vi "Serial Number Generator.vi"() -> (3 "UUT Serial #":string)   [LabVIEW 2018]
doc: "Generate a random serial number."
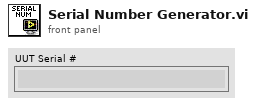
[diagram p1: front panel]
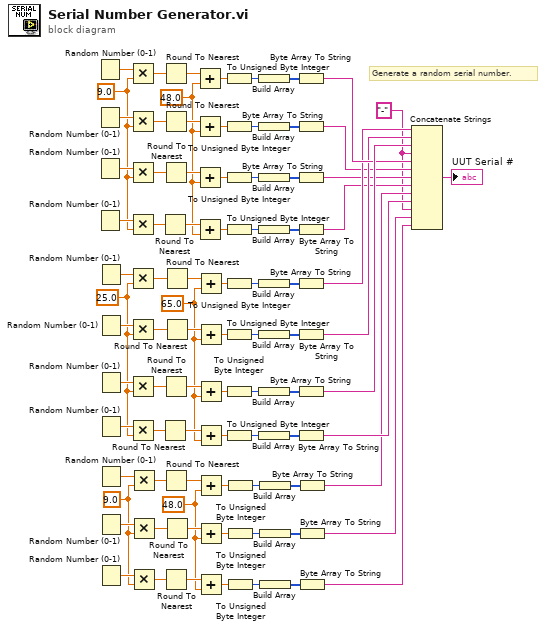
[diagram p0: block diagram]
diagram:
  w1 = 48.0
  w2 = 65.0
  w3 = 48.0
  w6 = 9.0
  w7 = 25.0
  w8 = 9.0
  w4 = "-" ("Substring")
  # "Generate a random serial number."
  n1 = Random Number (0-1)() -> (number: 0 to 1=w9:dbl)
  n2 = Random Number (0-1)() -> (number: 0 to 1=w54:dbl)
  n3 = Random Number (0-1)() -> (number: 0 to 1=w48:dbl)
  n4 = Random Number (0-1)() -> (number: 0 to 1=w42:dbl)
  n5 = Random Number (0-1)() -> (number: 0 to 1=w81:dbl)
  n6 = Random Number (0-1)() -> (number: 0 to 1=w68:dbl)
  n7 = Random Number (0-1)() -> (number: 0 to 1=w67:dbl)
  n8 = Random Number (0-1)() -> (number: 0 to 1=w57:dbl)
  n9 = Random Number (0-1)() -> (number: 0 to 1=w25:dbl)
  n10 = Random Number (0-1)() -> (number: 0 to 1=w30:dbl)
  n11 = Random Number (0-1)() -> (number: 0 to 1=w36:dbl)
  n12 = Multiply(x=w9, y=w8) -> (x*y=w80:dbl)
  n13 = Multiply(x=w54, y=w8) -> (x*y=w55:dbl)
  n14 = Multiply(x=w48, y=w8) -> (x*y=w49:dbl)
  n15 = Multiply(x=w42, y=w8) -> (x*y=w41:dbl)
  n16 = Multiply(x=w81, y=w7) -> (x*y=w79:dbl)
  n17 = Multiply(x=w68, y=w7) -> (x*y=w69:dbl)
  n18 = Multiply(x=w67, y=w7) -> (x*y=w66:dbl)
  n19 = Multiply(x=w57, y=w7) -> (x*y=w58:dbl)
  n20 = Multiply(x=w25, y=w6) -> (x*y=w26:dbl)
  n21 = Multiply(x=w30, y=w6) -> (x*y=w29:dbl)
  n22 = Multiply(x=w36, y=w6) -> (x*y=w35:dbl)
  n23 = Round To Nearest(number=w41) -> (nearest integer value=w17:dbl)
  n24 = Round To Nearest(number=w58) -> (nearest integer value=w13:dbl)
  n25 = Round To Nearest(number=w80) -> (nearest integer value=w20:dbl)
  n26 = Round To Nearest(number=w55) -> (nearest integer value=w19:dbl)
  n27 = Round To Nearest(number=w49) -> (nearest integer value=w18:dbl)
  n28 = Round To Nearest(number=w66) -> (nearest integer value=w14:dbl)
  n29 = Round To Nearest(number=w26) -> (nearest integer value=w12:dbl)
  n30 = Round To Nearest(number=w35) -> (nearest integer value=w10:dbl)
  n31 = Round To Nearest(number=w79) -> (nearest integer value=w16:dbl)
  n32 = Round To Nearest(number=w69) -> (nearest integer value=w15:dbl)
  n33 = Round To Nearest(number=w29) -> (nearest integer value=w11:dbl)
  n34 = Add(x=w20, y=w3) -> (x+y=w78:dbl)
  n35 = Add(x=w19, y=w3) -> (x+y=w56:dbl)
  n36 = Add(x=w18, y=w3) -> (x+y=w50:dbl)
  n37 = Add(x=w17, y=w3) -> (x+y=w40:dbl)
  n38 = Add(x=w16, y=w2) -> (x+y=w74:dbl)
  n39 = Add(x=w15, y=w2) -> (x+y=w73:dbl)
  n40 = Add(x=w14, y=w2) -> (x+y=w63:dbl)
  n41 = Add(x=w13, y=w2) -> (x+y=w62:dbl)
  n42 = Add(x=w12, y=w1) -> (x+y=w27:dbl)
  n43 = Add(x=w11, y=w1) -> (x+y=w28:dbl)
  n44 = Add(x=w10, y=w1) -> (x+y=w34:dbl)
  n45 = To Unsigned Byte Integer(number=w78) -> (unsigned 8bit integer=w83:u8)
  n46 = To Unsigned Byte Integer(number=w56) -> (unsigned 8bit integer=w52:u8)
  n47 = To Unsigned Byte Integer(number=w50) -> (unsigned 8bit integer=w46:u8)
  n48 = To Unsigned Byte Integer(number=w40) -> (unsigned 8bit integer=w43:u8)
  n49 = To Unsigned Byte Integer(number=w74) -> (unsigned 8bit integer=w76:u8)
  n50 = To Unsigned Byte Integer(number=w73) -> (unsigned 8bit integer=w71:u8)
  n51 = To Unsigned Byte Integer(number=w63) -> (unsigned 8bit integer=w65:u8)
  n52 = To Unsigned Byte Integer(number=w62) -> (unsigned 8bit integer=w60:u8)
  n53 = To Unsigned Byte Integer(number=w27) -> (unsigned 8bit integer=w23:u8)
  n54 = To Unsigned Byte Integer(number=w28) -> (unsigned 8bit integer=w32:u8)
  n55 = To Unsigned Byte Integer(number=w34) -> (unsigned 8bit integer=w38:u8)
  n56 = Build Array(w83) -> (w84:u8[])
  n57 = Build Array(w52) -> (w51:u8[])
  n58 = Build Array(w46) -> (w45:u8[])
  n59 = Build Array(w43) -> (w44:u8[])
  n60 = Build Array(w76) -> (w75:u8[])
  n61 = Build Array(w71) -> (w72:u8[])
  n62 = Build Array(w65) -> (w64:u8[])
  n63 = Build Array(w60) -> (w61:u8[])
  n64 = Build Array(w23) -> (w22:u8[])
  n65 = Build Array(w32) -> (w33:u8[])
  n66 = Build Array(w38) -> (w39:u8[])
  n67 = Byte Array To String(unsigned byte array=w84) -> (string=w82:string)
  n68 = Byte Array To String(unsigned byte array=w51) -> (string=w53:string)
  n69 = Byte Array To String(unsigned byte array=w45) -> (string=w47:string)
  n70 = Byte Array To String(unsigned byte array=w44) -> (string=w5:string)
  n71 = Byte Array To String(unsigned byte array=w75) -> (string=w77:string)
  n72 = Byte Array To String(unsigned byte array=w72) -> (string=w70:string)
  n73 = Byte Array To String(unsigned byte array=w64) -> (string=w85:string)
  n74 = Byte Array To String(unsigned byte array=w61) -> (string=w59:string)
  n75 = Byte Array To String(unsigned byte array=w22) -> (string=w24:string)
  n76 = Byte Array To String(unsigned byte array=w33) -> (string=w31:string)
  n77 = Byte Array To String(unsigned byte array=w39) -> (string=w37:string)
  n78 = Concatenate Strings(w77, w70, w85, w4, w82, w53, w47, w5, w24, w59, w4, w31, w37) -> (→"UUT Serial #":string)
